vi "funny average.vi"(10 "in":dbl[](array[numeric])) -> (2 "Out":dbl[](array[numeric]))   [LabVIEW 2020]
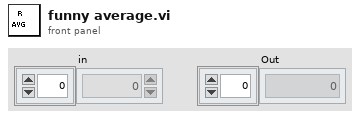
[diagram p1: front panel]
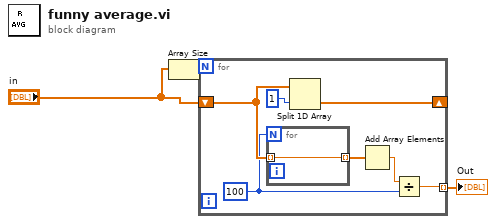
[diagram p0: block diagram]
diagram:
  n1 = Array Size(array="in") -> (size(s)=w3:i32)
  n2 = for {
    N: w3 -> [_]
    shift-right: [w8] -> _
    shift-left: "in" -> [w10]
    tunnel: [w4] -> w1 mode=indexing
    w5 = 100
    n3 = for {
      N: w5 -> [_]
      tunnel: w10 -> [w11] mode=indexing
      tunnel: [w11] -> w7 mode=indexing
    }
    n4 = Split 1D Array(array=w10, index=1) -> (second subarray=w8:dbl[])  [unwired: 1 out]
    n5 = Add Array Elements(numeric array=w7) -> (sum=w6:dbl)
    n6 = Divide(x=w6, y=w5) -> (x/y=w4:dbl)
  }
  "Out" <- w1
